vi "Write Load.vi"(8 "error in (no error)":errorcluster, 9 "Pic Width":dbl, 10 "CPU Load":dbl, 11 "CPU Bar in":refnum<class "CPU Bar.lvclass">) -> (0 "error out":errorcluster, 3 "CPU Bar out":refnum<class "CPU Bar.lvclass">)   [LabVIEW 2016, in "CPU Bar.lvclass"]
uses:
  CPU Bar.lvclass
  C:/Program Files (x86)/National Instruments/LabVIEW 2016/vi.lib/LIEF/Forms/Shape/Shape.lvclass
  CPU Bar.lvclass/CPU Bar.ctl
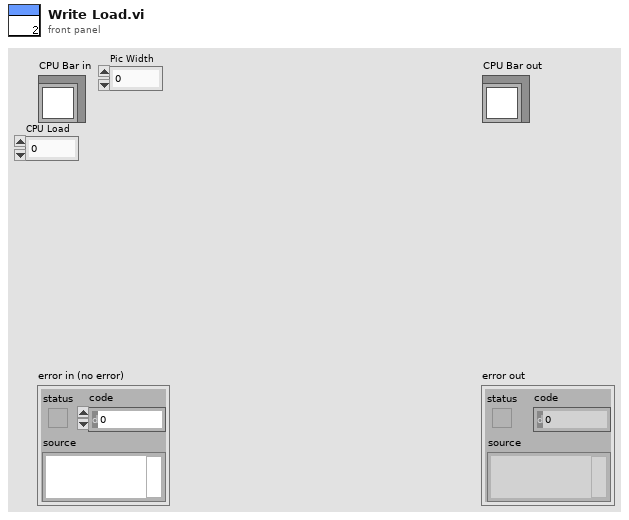
[diagram p1: front panel]
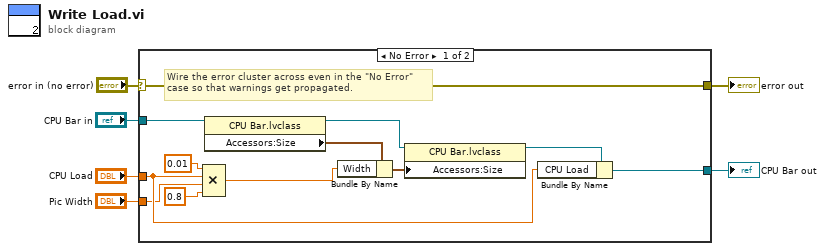
[diagram p0: block diagram]
diagram:
  n1 = case shown="No Error" "error in (no error)" {
    selector: "error in (no error)" -> [w18 w20]
    tunnel: [w18 w20] -> w5
    tunnel: [w9 w19] -> w3
    tunnel: "CPU Bar in" -> [w11 w19]
    tunnel: "CPU Load" -> [w8 _]
    tunnel: "Pic Width" -> [w7 _]
    frame No Error {
      # "Wire the error cluster across even in the \"No Error\"\ncase so that warnings get propagated."
      n2 = Compound Arithmetic op=MULTIPLY(0.01 ("value"), w8, w7, 0.8 ("value")) -> (w12:dbl)
      n3 = property class="CPU Bar.lvclass"(reference=w11) -> (reference out=w17:refnum<class "CPU Bar.lvclass">, "Accessors:Size"=w16:cluster{"Width":i32, "Height":i32})  [unwired: 1 in, 1 out]
      n4 = Bundle By Name(cluster=w16, "Width"=w12) -> (w15:cluster{"Width":i32, "Height":i32})
      n5 = property class="CPU Bar.lvclass"(reference=w17, "Accessors:Size"=w15) -> (reference out=w10:refnum<class "CPU Bar.lvclass">)  [unwired: 1 in, 1 out]
      n6 = Bundle By Name(cluster=w10, "CPU Load"=w8) -> (w9:refnum<class "CPU Bar.lvclass">)
    }
    frame Error {
    }
  }
  "error out" <- w5
  "CPU Bar out" <- w3
